vi "Get Rx Label Configuration.vi"(8 "error in":errorcluster, 10 "configuration string":string, 11 "port ref":T1 format="%.0x") -> (0 "error out":errorcluster, 2 "configuration string out":string, 3 "port ref out":T1 format="%.0x")   [LabVIEW 2020, in "Ballard ARINC 429 Hardware Configuration.lvlib"]
uses:
  Ballard ARINC 429 Hardware Configuration.lvlib
  <vilib>/NI VeriStand/Custom Device API/Custom Device Item Ref.ctl
  Constants.vi
  Scripting/Ballard/Ballard ARINC 429 Scripting.lvlib
  <vilib>/NI VeriStand/Custom Device API/Custom Device API.lvlib
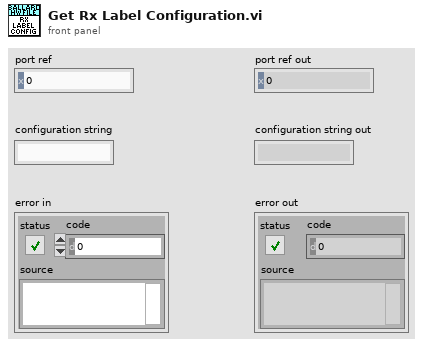
[diagram p1: front panel]
types:
  T1 = typedef "Custom Device API.lvlib/Custom Device Item Ref.ctl" = u64
  T2 = typedef "Label Properties.ctl" = cluster{"label (Dec)":T3, "SDI value":u8, "SDI enabled":bool}
  T3 = typedef "Label.ctl" = u8
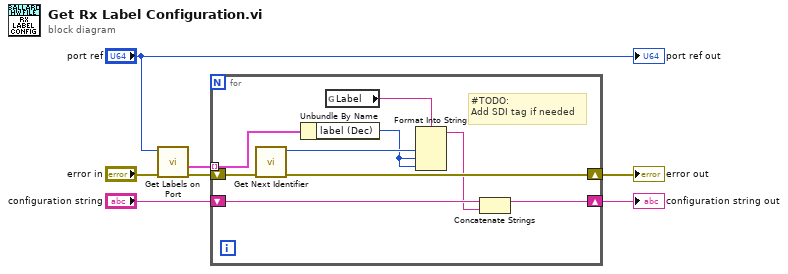
[diagram p0: block diagram]
diagram:
  n1 = call "Get Labels on Port.vi"("error in"="error in", "port in"="port ref") -> ("error out"=w3:errorcluster, "labels properties"=w7:T2[])  [unwired: 6 in, 2 out]
  n2 = for {
    tunnel: w7 -> [w16] mode=indexing
    shift-right: [w12] -> w5
    shift-left: "configuration string" -> [w9]
    shift-right: [w10] -> w2
    shift-left: w3 -> [w11]
    # "#TODO:\nAdd SDI tag if needed"
    n3 = call "Get Next Identifier.vi"("error in"=w11) -> ("error out"=w10:errorcluster, "ID"=w14:u32)  [unwired: 9 in]
    n4 = Unbundle By Name(w16) -> ("label (Dec)"=w13:T3)
    n5 = global read "Constants.vi" "Label"() -> (w15:string)
    n6 = Format Into String(format string=w15, w14, w13, w13) -> (resulting string=w8:string)  [unwired: 2 in, 1 out]
    n7 = Concatenate Strings(w9, w8) -> (w12:string)
  }
  "error out" <- w2
  "configuration string out" <- w5
  "port ref out" <- "port ref"
